vi "Read (Multiple Points).vi"(8 "error in (no error)":errorcluster, 9 "Timeout (10000 ms)":i32=10000 format="%#.6g", 10 "Sample Count (1)":i32=1, 11 "VISA resource name":refnum<visa-resource-name>) -> (0 "error out":errorcluster, 2 "Measurements":dbl[][](array[numeric]), 3 "VISA resource name out":refnum<visa-resource-name>)   [LabVIEW 2024]
doc: "Reads and returns multiple measurements from the instrument. Use this VI when you want to take multiple measurements using an immediate trigger. Use the low-level VIs for other triggering options."
uses:
  EFmeter.lvlib
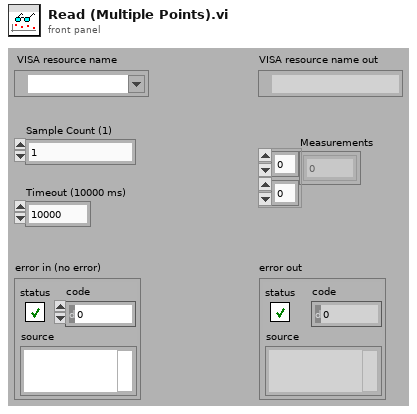
[diagram p1: front panel]
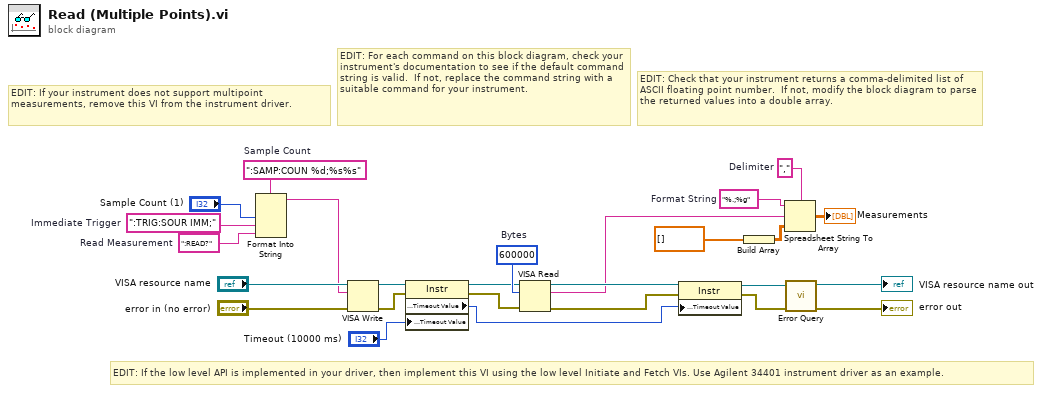
[diagram p0: block diagram]
diagram:
  w5 = ","  # Delimiter
  w6 = "%.;%g"  # Format String
  w7 = ":TRIG:SOUR IMM;"  # Immediate Trigger
  w11 = ":SAMP:COUN %d;%s%s"  # Sample Count
  w8 = ":READ?"  # Read Measurement
  w26 = u32 600000  # Bytes
  # "EDIT: If the low level API is implemented in your driver, then implement this VI using the low level Initiate and Fetch VIs. Use Agilent 34401 instrument driver as an example."
  # "EDIT: If your instrument does not support multipoint measurements, remove this VI from the instrument driver."
  # "EDIT: Check that your instrument returns a comma-delimited list of ASCII floating point number.  If not, modify the block diagram to parse the returned values into a double array."
  # "EDIT: For each command on this block diagram, check your instrument's documentation to see if the default command string is valid.  If not, replace the command string with a suitable command for your instrument."
  n1 = Format Into String(format string=w11, "Sample Count (1)", w7, w8) -> (resulting string=w9:string)  [unwired: 2 in, 1 out]
  n2 = VISA Write(VISA resource name="VISA resource name", write buffer=w9, error in (no error)="error in (no error)") -> (VISA resource name out=w21:refnum<visa-resource-name>, error out=w20:errorcluster)  [unwired: 1 out]
  n3 = property on="Property Node" class="Instr"(reference=w21, error in=w20, "General Settings:Timeout Value"="Timeout (10000 ms)") -> (reference out=w19:refnum<visa-resource-name>, error out=w18:errorcluster, "General Settings:Timeout Value"=w12:u32)
  n4 = VISA Read(VISA resource name=w19, byte count=w26, error in (no error)=w18) -> (VISA resource name out=w16:refnum<visa-resource-name>, read buffer=w1:string, error out=w14:errorcluster)  [unwired: 1 out]
  n5 = property on="Property Node" class="Instr"(reference=w16, error in=w14, "General Settings:Timeout Value"=w12) -> (reference out=w15:refnum<visa-resource-name>, error out=w13:errorcluster)
  n6 = Build Array(dbl[] []) -> (w4:dbl[][])
  n7 = Spreadsheet String To Array(delimiter (Tab)=w5, format string=w6, spreadsheet string=w1, array type (2D Dbl)=w4) -> (array=→"Measurements":dbl[][])
  n8 = call "Error Query.vi"("error in (no error)"=w13, "VISA resource name"=w15) -> ("error out"=→"error out":errorcluster, "VISA resource name out"=→"VISA resource name out":refnum<visa-resource-name>)  [unwired: 6 in, 2 out]
